vi "close tdms.vi"(8 "error in (no error)":errorcluster, 11 "device_type in":refnum<class "device_type.lvclass">) -> (0 "error out":errorcluster, 3 "device_type out":refnum<class "device_type.lvclass">)   [LabVIEW 2021, in "device_type.lvclass"]
uses:
  device_type.lvclass
  device_type.lvclass/device_type.ctl
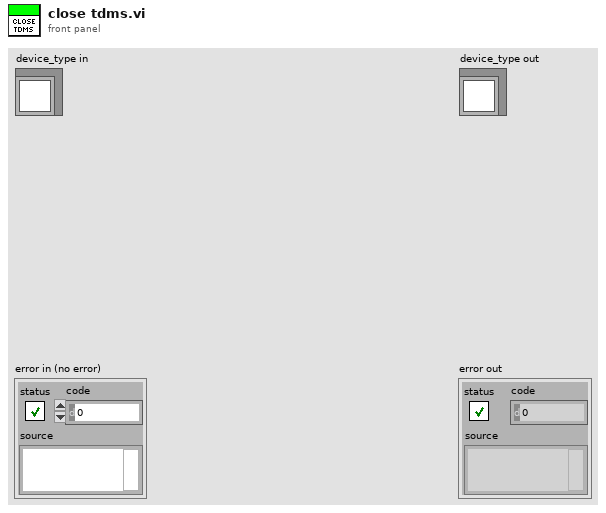
[diagram p1: front panel]
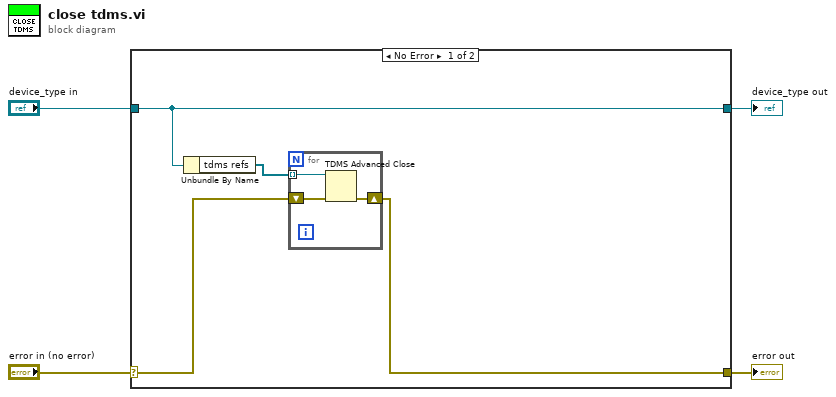
[diagram p0: block diagram]
diagram:
  n1 = case shown="No Error" "error in (no error)" {
    selector: "error in (no error)" -> [w6 w13]
    tunnel: [w5 w13] -> w3
    tunnel: [w8 w12] -> w1
    tunnel: "device_type in" -> [w8 w12]
    frame No Error {
      n2 = Unbundle By Name(w8) -> ("tdms refs"=w7:refnum<k34>[])
      n3 = for {
        shift-right: [w10] -> w5
        shift-left: w6 -> [w11]
        tunnel: w7 -> [w9] mode=indexing
        n4 = TDMS Advanced Close(8:w11, 11:w9) -> (0:w10:errorcluster)  [unwired: 2 in, 1 out]
      }
    }
    frame Error {
    }
  }
  "error out" <- w3
  "device_type out" <- w1
